vi "test_mapping_coordinates.vi"(7 "Parameters":T1, 8 "Error In":errorcluster, 9 "ROI":T2, 10 "original image name":string, 11 "File Path":path) -> (0 "Error Out":errorcluster, 3 "Parameters Out":T1)   [LabVIEW 2019]
uses:
  image_property_cluster_typedef.ctl
  xi_angles_enum_typedef.ctl
  parameters_cluster_typedef.ctl
  tune_c_parameter_states_enum_typedef.ctl
  <vilib>/vision/NI_Vision_Development_Module.lvlib
panel:
  out "ROI Out":T2
  in  "Xi":T3
  in  "Operator Value":sgl format="%.2f"
  in  "Operator":T4(ring)
  out "Image Properties":T5
  in  "Done":bool
  in  "Frame":i32(slide) min=0 max=19 step=1 scale=0.0..11.0
  out "Projected Boundaries":T6(plugin-control)
  out "Original Image":T6(plugin-control)
  # "Tune Parameters"
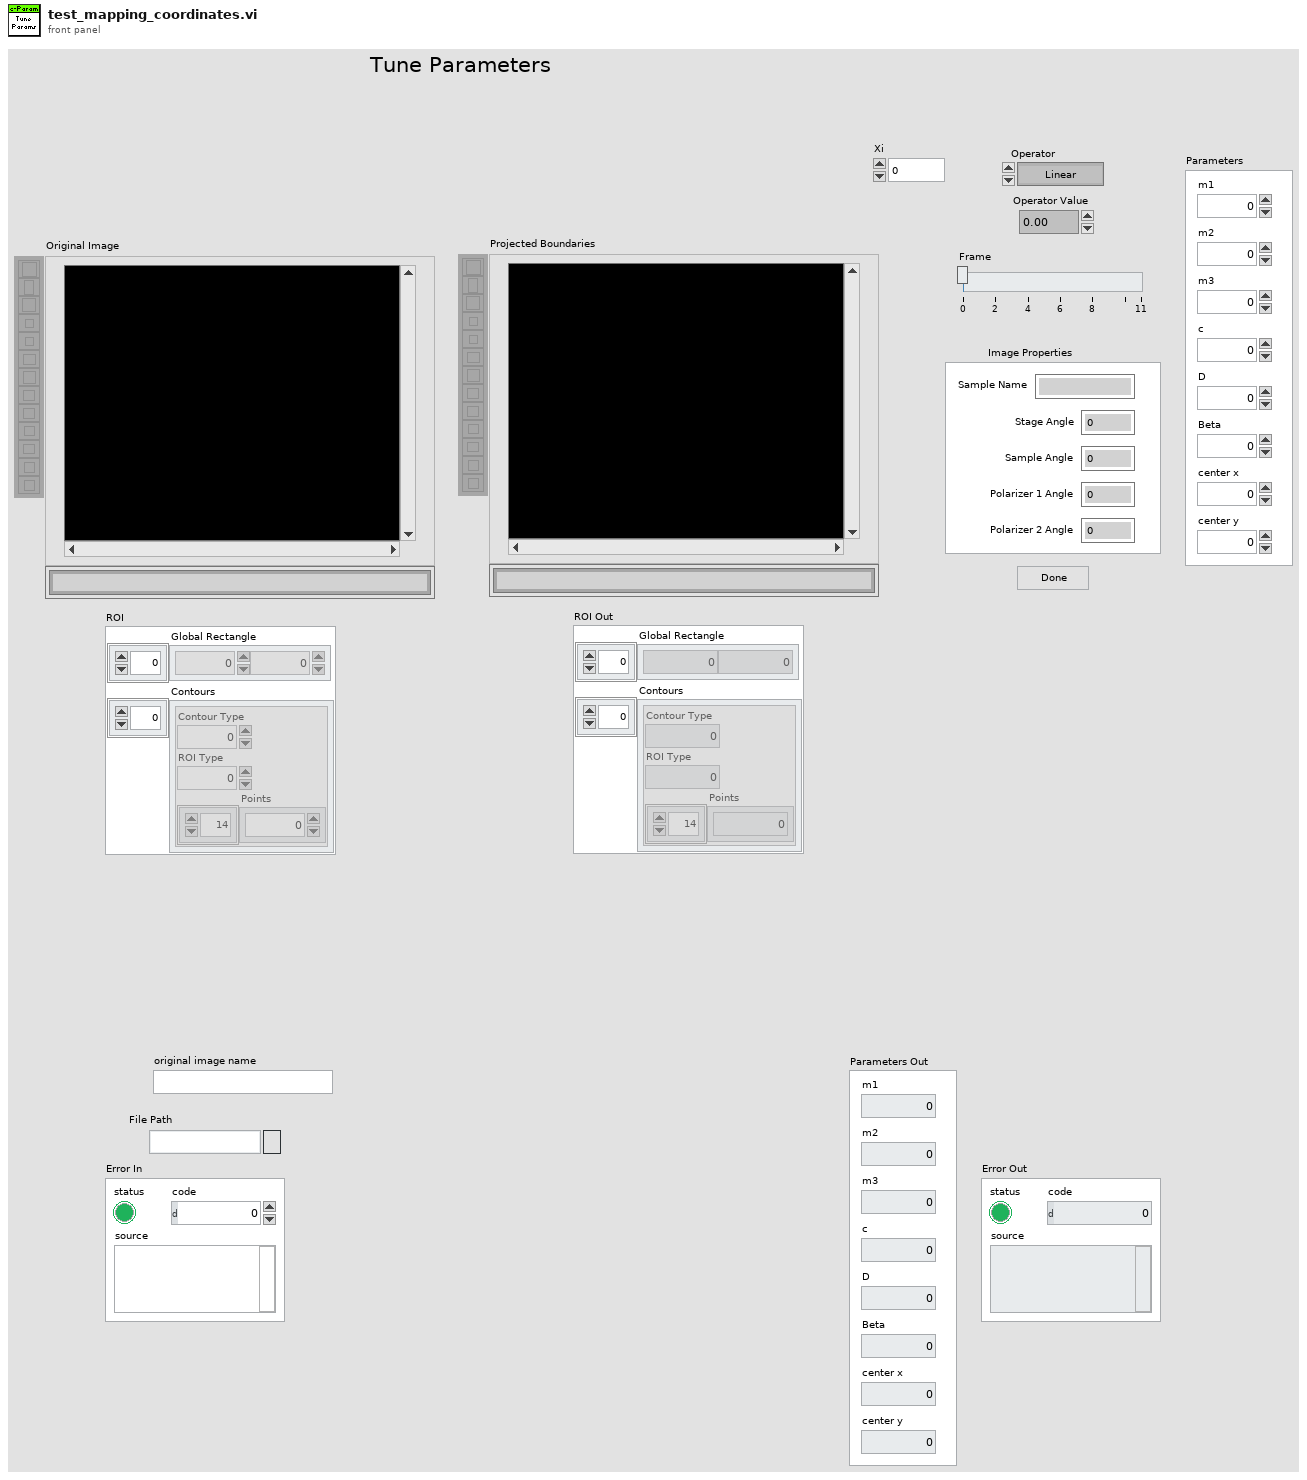
[diagram p1: front panel]
types:
  T1 = typedef "parameters_cluster_typedef.ctl" = cluster{"m1":dbl, "m2":dbl, "m3":dbl, "c":dbl, "D":dbl, "Beta":dbl, "center x":dbl, "center y":dbl}
  T2 = cluster{"Global Rectangle":i32[], "Contours":cluster{"Contour Type":u32, "ROI Type":u32, "Points":i32[]}[]}
  T3 = typedef "xi_angles_enum_typedef.ctl" = enum16{"0", "45"}
  T4 = enum32{"Linear", "Log", "Exp", "Square", "Square root", "Power X", "Power 1/X"}
  T5 = typedef "image_property_cluster_typedef.ctl" = cluster{"Stage Angle":dbl, "Sample Angle":dbl, "Polarizer 1 Angle":dbl, "Polarizer 2 Angle":dbl, "Sample Name":string}
  T6 = typedef "IMAQ Image.ctl" = refnum<image>
  T7 = typedef "tune_c_parameter_states_enum_typedef.ctl" = enum16{"Shutdown", "Wait", "Initialize", "Plot", "Change Sequence"}
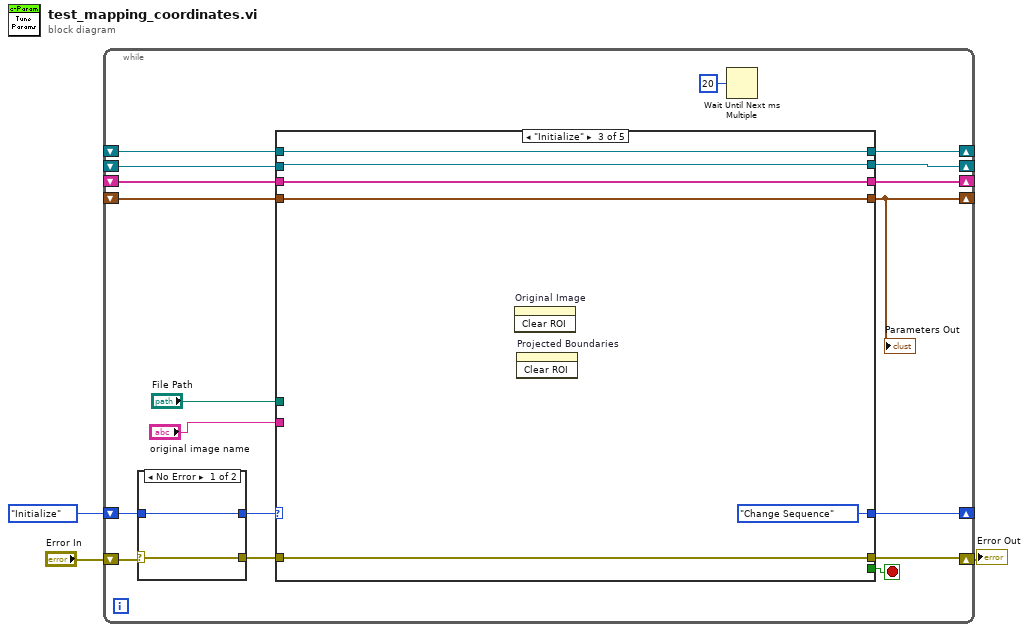
[diagram p0: block diagram]
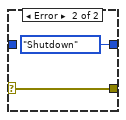
[diagram p2: hidden frame]
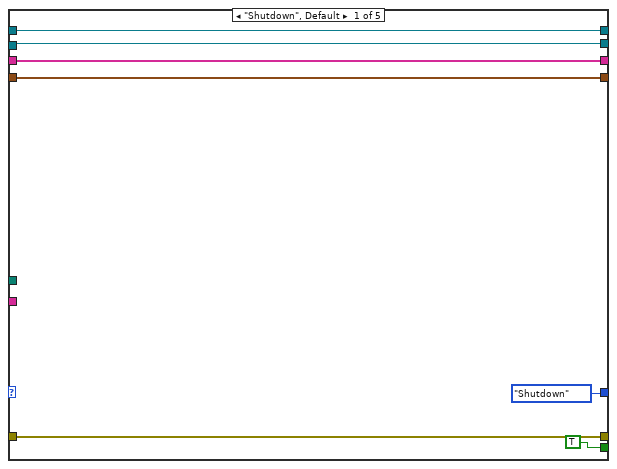
[diagram p3: hidden frame]
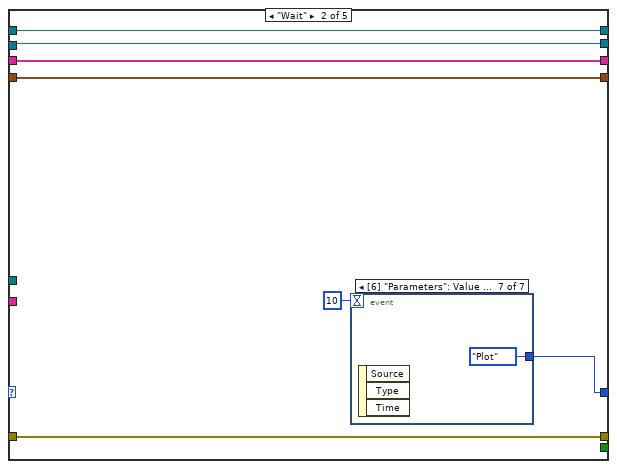
[diagram p4: hidden frame]
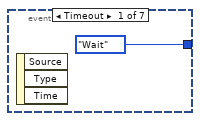
[diagram p5: hidden frame]
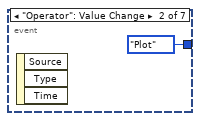
[diagram p6: hidden frame]
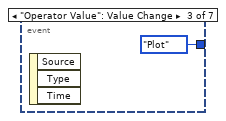
[diagram p7: hidden frame]
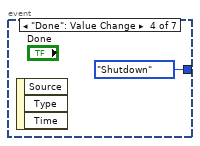
[diagram p8: hidden frame]
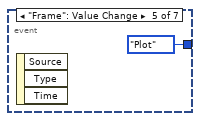
[diagram p9: hidden frame]
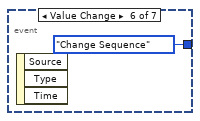
[diagram p10: hidden frame]
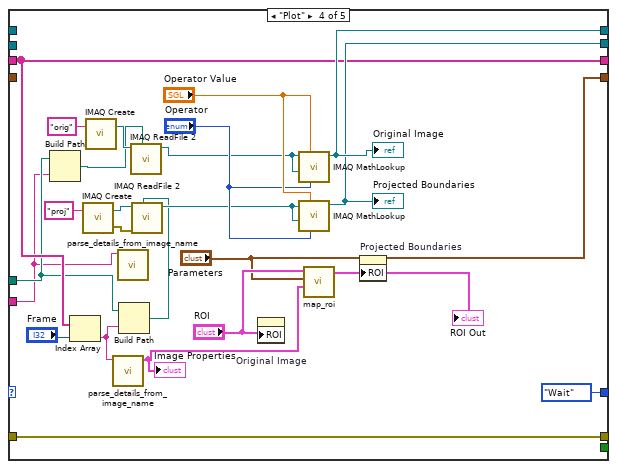
[diagram p11: hidden frame]
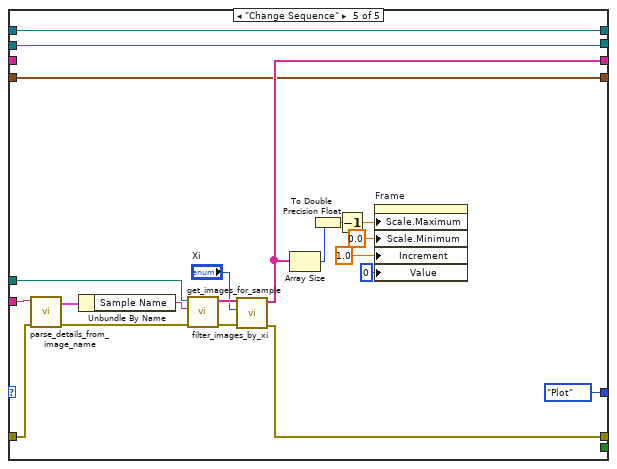
[diagram p12: hidden frame]
diagram:
  n1 = while {
    shift-right: [w16] -> w1
    shift-left: "Error In" -> [w21]
    shift-right: [w17] -> _
    shift-left: tune_c_parameter_states_enum_typedef."Initialize" -> [w18]
    shift-right: [w11] -> _
    shift-left: _ -> [w10]
    shift-right: [w9] -> _
    shift-left: _ -> [w8]
    shift-right: [w7] -> _
    shift-left: _ -> [w6]
    shift-right: [w5] -> _
    shift-left: _ -> [w4]
    stop <- w15 stop-if-true
    n2 = case shown="No Error" w21 {
      selector: w21 -> [w23 w25]
      tunnel: [w23 w25] -> w20
      tunnel: [w22 tune_c_parameter_states_enum_typedef."Shutdown"] -> w19
      tunnel: w18 -> [w22 _]
      frame No Error {
      }
      frame Error {
      }
    }
    n3 = case shown="\"Initialize\"" w19 {
      tunnel: w20 -> [w31 w39 w48 w75 w83]
      tunnel: [tune_c_parameter_states_enum_typedef."Shutdown" w37 tune_c_parameter_states_enum_typedef."Change Sequence" tune_c_parameter_states_enum_typedef."Wait" tune_c_parameter_states_enum_typedef."Plot"] -> w17
      tunnel: [w31 w39 w48 w75 w81] -> w16
      tunnel: [TRUE _ _ _ _] -> w15
      tunnel: "File Path" -> [_ _ _ w63 w86]
      tunnel: "original image name" -> [_ _ _ w56 w89]
      tunnel: [w29 w36 w51 w67 w85] -> w11
      tunnel: w10 -> [w29 w36 w51 _ w85]
      tunnel: [w28 w35 w50 w66 w84] -> w9
      tunnel: w8 -> [w28 w35 w50 _ w84]
      tunnel: [w27 w34 w49 w64 w80] -> w7
      tunnel: w6 -> [w27 w34 w49 w64 _]
      tunnel: [w26 w33 w47 "Parameters" w77] -> w5
      tunnel: w4 -> [w26 w33 w47 _ w77]
      frame "Shutdown", Default {
      }
      frame "Wait" {
        n4 = event shown="[6] \"Parameters\": Value Change" {
          selector: _ -> [_ _ _ _ _ _ _]
          dyn-events: _ -> [_ _ _ _ _ _ _]
          timeout: 10 -> [_ _ _ _ _ _ _]
          tunnel: [tune_c_parameter_states_enum_typedef."Wait" tune_c_parameter_states_enum_typedef."Plot" tune_c_parameter_states_enum_typedef."Plot" tune_c_parameter_states_enum_typedef."Shutdown" tune_c_parameter_states_enum_typedef."Plot" tune_c_parameter_states_enum_typedef."Change Sequence" tune_c_parameter_states_enum_typedef."Plot"] -> w37
          event Timeout {
            n5 = event-data() -> ()  [unwired: 1 in, 3 out]
          }
          event "Operator": Value Change {
            n6 = event-data() -> ()  [unwired: 1 in, 3 out]
          }
          event "Operator Value": Value Change {
            n7 = event-data() -> ()  [unwired: 1 in, 3 out]
          }
          event "Done": Value Change {
            n8 = event-data() -> ()  [unwired: 1 in, 3 out]
          }
          event "Frame": Value Change {
            n9 = event-data() -> ()  [unwired: 1 in, 3 out]
          }
          event Value Change {
            n10 = event-data() -> ()  [unwired: 1 in, 3 out]
          }
          event Value Change {
            n11 = event-data() -> ()  [unwired: 1 in, 3 out]
          }
        }
      }
      frame "Initialize" {
        n12 = invoke on="Original Image" class="ImageControl" method="Clear ROI"() -> ()  [unwired: 3 in, 3 out]
        n13 = invoke on="Projected Boundaries" class="ImageControl" method="Clear ROI"() -> ()  [unwired: 3 in, 3 out]
      }
      frame "Plot" {
        n14 = Build Path(base path=w63, name or relative path=w56) -> (appended path=w70:path)
        n15 = Index Array(array=w64, index="Frame") -> (element=w58:string)
        n16 = call "IMAQ Create"("Image Name"="proj") -> ("New Image"=w62:T6, "error out"=w61:errorcluster)  [unwired: 4 in]
        n17 = call "IMAQ Create"("Image Name"="orig") -> ("New Image"=w71:T6)  [unwired: 4 in, 1 out]
        n18 = call "parse_details_from_image_name.vi"("Image Name"=w58) -> ("Image Properties"=w54:T5)  [unwired: 9 in, 1 out]
        "Image Properties" <- w54
        n19 = call "parse_details_from_image_name.vi"("Image Name"=w56) -> ()  [unwired: 9 in, 2 out]
        n20 = Build Path(base path=w63, name or relative path=w58) -> (appended path=w59:path)
        n21 = call "IMAQ ReadFile 2"("File Path"=w70, "Image"=w71) -> ("Image Out"=w69:T6)  [unwired: 5 in, 4 out]
        n22 = call "IMAQ ReadFile 2"("File Path"=w59, "error in (no error)"=w61, "Image"=w62) -> ("Image Out"=w68:T6)  [unwired: 4 in, 4 out]
        n23 = property on="Original Image" class="ImageControl"("ROI"="ROI") -> ()  [unwired: 2 in, 2 out]
        n24 = call "IMAQ MathLookup"("Operator"="Operator", "X Value"="Operator Value", "Image Dst"=w69, "Image Src"=w69) -> ("Image Dst Out"=w67:T6)  [unwired: 6 in, 1 out]
        "Original Image" <- w67
        n25 = call "IMAQ MathLookup"("Operator"="Operator", "X Value"="Operator Value", "Image Dst"=w68, "Image Src"=w68) -> ("Image Dst Out"=w66:T6)  [unwired: 6 in, 1 out]
        "Projected Boundaries" <- w66
        n26 = call "map_roi.vi"("Image Properties"=w54, "Parameters"="Parameters", "ROI In"="ROI") -> ("ROI Out"=w55:T2)  [unwired: 7 in, 1 out]
        "ROI Out" <- w55
        n27 = property on="Projected Boundaries" class="ImageControl"("ROI"=w55) -> ()  [unwired: 2 in, 2 out]
      }
      frame "Change Sequence" {
        n28 = call "parse_details_from_image_name.vi"("Error In"=w83, "Image Name"=w89) -> ("Error Out"=w82:errorcluster, "Image Properties"=w88:T5)  [unwired: 8 in]
        n29 = Unbundle By Name(w88) -> ("Sample Name"=w87:string)
        n30 = call "get_images_for_sample.vi"("Error In"=w82, "Sample"=w87, "File Path"=w86) -> ("Error Out"=w96:errorcluster, "Image Names"=w95:string[])  [unwired: 7 in]
        n31 = call "filter_images_by_xi.vi"("Error In"=w96, "Xi"="Xi", "Image Names"=w95) -> ("Error Out"=w81:errorcluster, "Filtered Image Names"=w80:string[])  [unwired: 7 in]
        n32 = Array Size(array=w80) -> (size(s)=w93:i32)
        n33 = To Double Precision Float(number=w93) -> (double precision float=w79:dbl)
        n34 = Decrement(x=w79) -> (x-1=w78:dbl)
        n35 = property on="Frame" class="Slide (strict)"("Scale.Maximum"=w78, "Scale.Minimum"=0.0 ("Scale.Range:Minimum"), "Increment"=1.0 ("Data Entry Limits:Increment"), "Value"=0 ("Frame")) -> ()  [unwired: 2 in, 2 out]
      }
    }
    "Parameters Out" <- w5
    n36 = Wait Until Next ms Multiple(millisecond multiple=u32 20) -> ()  [unwired: 1 out]
  }
  "Error Out" <- w1
